vi "Auton_S2_Left_Switch.vi"   [LabVIEW 2017]
uses:
  <vilib>/Rock Robotics/WPI/Utilities/WPI_GetSetVariantRefNum.vi
  Robot Global Data.vi
  <vilib>/Rock Robotics/WPI/RobotDrive/WPI_RobotDriveArcadeDrive_Standard(NoSaturation).vi
types:
  T1 = typedef "WPI_RobotDriveDevRef.ctl" = cluster{"DevStatus":errorcluster, "Motors[]":T2[], "Square Inputs":bool, "Max Output":dbl}
  T2 = typedef "WPI_MotorControlDeviceRef.ctl" = cluster{"DeviceStatus":errorcluster, "Type":T3, "PWM":cluster{"PWM Channel":T4, "DeadBand":T5}, "CAN":cluster{"Device Number":u8, "SetOutput VI Ref":variant, "GetOutput VI Ref":variant, "Enable VI Ref":variant, "Disable VI Ref":variant, "Data":variant}, "Invert":bool, "DIO PWM":cluster{"PWM \"Enable\" Channel":T4, "DIOChannel":T6, "PWM Rate":dbl}}
  T3 = typedef "WPI_MotorControlType.ctl" = enum16{"PWM", "CAN", "DIO PWM"}
  T4 = typedef "FPGA_DIOPWMChannel.ctl" = enum8{"PWM 0", "PWM 1", "PWM 2", "PWM 3", "PWM 4", "PWM 5", "PWM 6", "PWM 7", "PWM 8", "PWM 9", "PWM MXP 0", "PWM MXP 1", "PWM MXP 2", "PWM MXP 3", "PWM MXP 4", "PWM MXP 5", "PWM MXP 6", "PWM MXP 7", "PWM MXP 8", "PWM MXP 9", "Invalid"}
  T5 = typedef "WPI_PWMDeadband.ctl" = cluster{"Name":string, "maxPositivePwm":i32, "minPositivePwm":i32, "centerPwm":i32, "maxNegativePwm":i32, "minNegativePwm":i32, "angularRange":u16}
  T6 = typedef "FPGA_DIOChannel.ctl" = enum8{"DIO 0", "DIO 1", "DIO 2", "DIO 3", "DIO 4", "DIO 5", "DIO 6", "DIO 7", "DIO 8", "DIO 9", "DIO MXP 0", "DIO MXP 1", "DIO MXP 2", "DIO MXP 3", "DIO MXP 4", "DIO MXP 5", "DIO MXP 6", "DIO MXP 7", "DIO MXP 8", "DIO MXP 9", "DIO MXP 10", "DIO MXP 11", "DIO MXP 12", "DIO MXP 13", "DIO MXP 14", "DIO MXP 15", "SPI Port CS1", "SPI Port CS2", "SPI Port CS3", "SPI Port MISO", "SPI Port MOSI", "Invalid"}
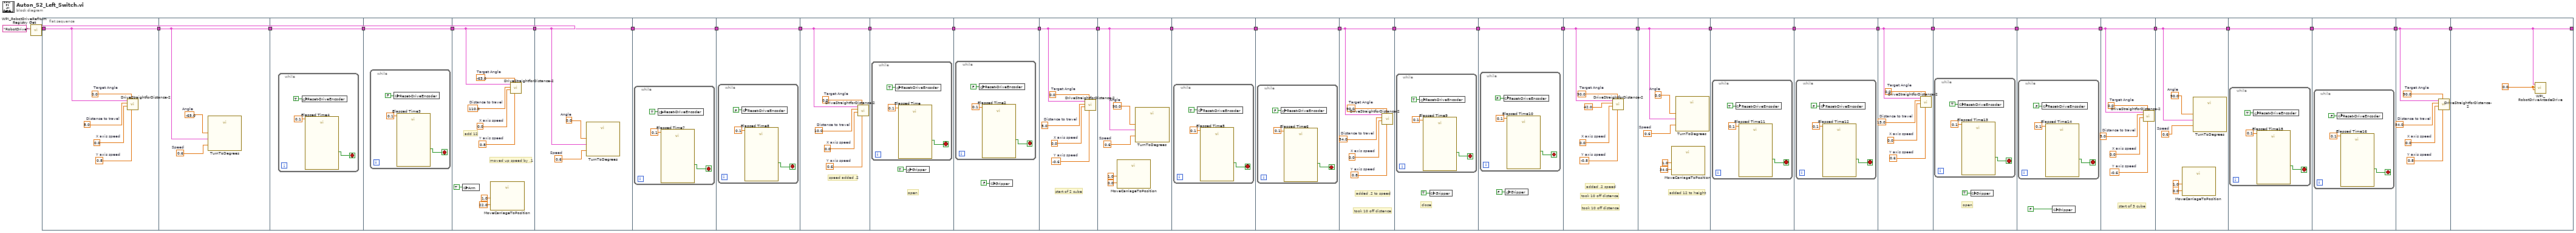
[diagram p0: block diagram]
diagram:
  n1 = call <vilib>:"WPI_RobotDriveRefNum Registry Get.vi"("refnum name"="RobotDrive") -> ("RobotDriveDevRef"=w31:T1)  [unwired: 9 in, 1 out]
  n2 = flat-sequence {
    tunnel: [w37] -> w28
    tunnel: w31 -> [w37]
    tunnel: w28 -> [w39]
    tunnel: [w39] -> w27
    tunnel: w27 -> [w41]
    tunnel: [w41] -> w29
    tunnel: w29 -> [w45]
    tunnel: [w45] -> w30
    tunnel: [w56] -> w26
    tunnel: w30 -> [w56]
    tunnel: w26 -> [w57]
    tunnel: [w57] -> w25
    tunnel: w25 -> [w60]
    tunnel: [w60] -> w24
    tunnel: w24 -> [w64]
    tunnel: [w64] -> w23
    tunnel: w23 -> [w68]
    tunnel: [w68] -> w22
    tunnel: w22 -> [w74]
    tunnel: [w74] -> w21
    tunnel: w21 -> [w79]
    tunnel: [w79] -> w20
    tunnel: w20 -> [w83]
    tunnel: [w83] -> w19
    tunnel: w19 -> [w90]
    tunnel: [w90] -> w18
    tunnel: w18 -> [w93]
    tunnel: [w93] -> w17
    tunnel: w17 -> [w97]
    tunnel: [w97] -> w16
    tunnel: w16 -> [w101]
    tunnel: [w101] -> w14
    tunnel: w14 -> [w107]
    tunnel: [w107] -> w13
    tunnel: w13 -> [w112]
    tunnel: [w112] -> w12
    tunnel: w12 -> [w116]
    tunnel: [w116] -> w15
    tunnel: w15 -> [w123]
    tunnel: [w123] -> w11
    tunnel: w11 -> [w126]
    tunnel: [w126] -> w10
    tunnel: w10 -> [w130]
    tunnel: [w130] -> w9
    tunnel: w9 -> [w134]
    tunnel: [w134] -> w8
    tunnel: w8 -> [w140]
    tunnel: [w140] -> w7
    tunnel: w7 -> [w145]
    tunnel: [w145] -> w6
    tunnel: w6 -> [w149]
    tunnel: [w149] -> w5
    tunnel: w5 -> [w154]
    tunnel: [w154] -> w4
    tunnel: w4 -> [w159]
    tunnel: [w159] -> w3
    tunnel: w3 -> [w163]
    tunnel: [w163] -> w2
    tunnel: w2 -> [w167]
    tunnel: [w167] -> w1
    tunnel: [w172] -> _
    tunnel: w1 -> [w172]
    frame #0 {
      w33 = 0.0  # Target Angle
      w34 = 0.8  # Y axis speed
      w35 = 0.0  # X axis speed
      w36 = 5.0  # Distance to travel
      n3 = call "DriveStraightforDistance-2.vi"("Y axis speed"=w34, "Target Angle"=w33, "X axis speed"=w35, "Distance to travel"=w36, "RobotDriveDevRef"=w37) -> ()  [unwired: 7 in]
    }
    frame #1 {
      w38 = -65.0  # Angle
      w40 = 0.6  # Speed
      n4 = call "TurnToDegrees.vi"("Speed"=w40, "RobotDriveDevRef"=w39, "Angle"=w38) -> ()  [unwired: 9 in]
    }
    frame #2 {
      n5 = while {
        stop <- w44 stop-if-true
        n6 = global write "Robot Global Data.vi" "Reset-DriveEncoder"(TRUE ("Reset-DriveEncoder")) -> ()
        n7 = call "Elapsed Time4"("Time Target (s)"=0.1) -> ("Time has Elapsed"=w44:bool)  [unwired: 11 in, 7 out]
      }
    }
    frame #3 {
      n8 = while {
        stop <- w48 stop-if-true
        n9 = global write "Robot Global Data.vi" "Reset-DriveEncoder"(FALSE ("Reset-DriveEncoder")) -> ()
        n10 = call "Elapsed Time3"("Time Target (s)"=0.1) -> ("Time has Elapsed"=w48:bool)  [unwired: 11 in, 7 out]
      }
    }
    frame #4 {
      w52 = -63.0  # Target Angle
      w53 = 0.8  # Y axis speed
      w54 = 0.0  # X axis speed
      w55 = 110.0  # Distance to travel
      # "add 12"
      # "moved up speed by .1"
      n11 = global write "Robot Global Data.vi" "Arm"(TRUE ("Arm")) -> ()
      n12 = call "MoveCarriageToPosition.vi"("Lift Speed"=1.0, "Target Height"=22.0) -> ()  [unwired: 10 in]
      n13 = call "DriveStraightforDistance-2.vi"("Y axis speed"=w53, "Target Angle"=w52, "X axis speed"=w54, "Distance to travel"=w55, "RobotDriveDevRef"=w56) -> ()  [unwired: 7 in]
    }
    frame #5 {
      w58 = 0.0  # Angle
      w59 = 0.6  # Speed
      n14 = call "TurnToDegrees.vi"("Speed"=w59, "RobotDriveDevRef"=w57, "Angle"=w58) -> ()  [unwired: 9 in]
    }
    frame #6 {
      n15 = while {
        stop <- w63 stop-if-true
        n16 = global write "Robot Global Data.vi" "Reset-DriveEncoder"(TRUE ("Reset-DriveEncoder")) -> ()
        n17 = call "Elapsed Time7"("Time Target (s)"=0.1) -> ("Time has Elapsed"=w63:bool)  [unwired: 11 in, 7 out]
      }
    }
    frame #7 {
      n18 = while {
        stop <- w67 stop-if-true
        n19 = global write "Robot Global Data.vi" "Reset-DriveEncoder"(FALSE ("Reset-DriveEncoder")) -> ()
        n20 = call "Elapsed Time8"("Time Target (s)"=0.1) -> ("Time has Elapsed"=w67:bool)  [unwired: 11 in, 7 out]
      }
    }
    frame #8 {
      w69 = 0.0  # Target Angle
      w70 = 0.6  # Y axis speed
      w71 = 0.0  # X axis speed
      w72 = 10.0  # Distance to travel
      # "speed added .2"
      n21 = call "DriveStraightforDistance-2.vi"("Y axis speed"=w70, "Target Angle"=w69, "X axis speed"=w71, "Distance to travel"=w72, "RobotDriveDevRef"=w68) -> ()  [unwired: 7 in]
    }
    frame #9 {
      # "open"
      n22 = while {
        stop <- w77 stop-if-true
        n23 = global write "Robot Global Data.vi" "Reset-DriveEncoder"(TRUE ("Reset-DriveEncoder")) -> ()
        n24 = call "Elapsed Time"("Time Target (s)"=0.1) -> ("Time has Elapsed"=w77:bool)  [unwired: 11 in, 7 out]
      }
      n25 = global write "Robot Global Data.vi" "Gripper"(TRUE ("Gripper")) -> ()
    }
    frame #10 {
      n26 = while {
        stop <- w82 stop-if-true
        n27 = global write "Robot Global Data.vi" "Reset-DriveEncoder"(FALSE ("Reset-DriveEncoder")) -> ()
        n28 = call "Elapsed Time2"("Time Target (s)"=0.1) -> ("Time has Elapsed"=w82:bool)  [unwired: 11 in, 7 out]
      }
      n29 = global write "Robot Global Data.vi" "Gripper"(FALSE ("Gripper")) -> ()
    }
    frame #11 {
      w84 = 0.0  # Target Angle
      w85 = -0.6  # Y axis speed
      w86 = 0.0  # X axis speed
      w87 = 5.0  # Distance to travel
      # "start of 2 cube"
      n30 = call "DriveStraightforDistance-2.vi"("Y axis speed"=w85, "Target Angle"=w84, "X axis speed"=w86, "Distance to travel"=w87, "RobotDriveDevRef"=w83) -> ()  [unwired: 7 in]
    }
    frame #12 {
      w91 = 90.0  # Angle
      w92 = 0.6  # Speed
      n31 = call "MoveCarriageToPosition.vi"("Lift Speed"=1.0, "Target Height"=0.0) -> ()  [unwired: 10 in]
      n32 = call "TurnToDegrees.vi"("Speed"=w92, "RobotDriveDevRef"=w90, "Angle"=w91) -> ()  [unwired: 9 in]
    }
    frame #13 {
      n33 = while {
        stop <- w96 stop-if-true
        n34 = global write "Robot Global Data.vi" "Reset-DriveEncoder"(TRUE ("Reset-DriveEncoder")) -> ()
        n35 = call "Elapsed Time5"("Time Target (s)"=0.1) -> ("Time has Elapsed"=w96:bool)  [unwired: 11 in, 7 out]
      }
    }
    frame #14 {
      n36 = while {
        stop <- w100 stop-if-true
        n37 = global write "Robot Global Data.vi" "Reset-DriveEncoder"(FALSE ("Reset-DriveEncoder")) -> ()
        n38 = call "Elapsed Time6"("Time Target (s)"=0.1) -> ("Time has Elapsed"=w100:bool)  [unwired: 11 in, 7 out]
      }
    }
    frame #15 {
      w102 = 90.0  # Target Angle
      w103 = 0.8  # Y axis speed
      w104 = 0.0  # X axis speed
      w105 = 54.0  # Distance to travel
      # "took 10 off distence"
      # "added .2 to speed"
      n39 = call "DriveStraightforDistance-2.vi"("Y axis speed"=w103, "Target Angle"=w102, "X axis speed"=w104, "Distance to travel"=w105, "RobotDriveDevRef"=w101) -> ()  [unwired: 7 in]
    }
    frame #16 {
      # "close"
      n40 = while {
        stop <- w110 stop-if-true
        n41 = global write "Robot Global Data.vi" "Reset-DriveEncoder"(TRUE ("Reset-DriveEncoder")) -> ()
        n42 = call "Elapsed Time9"("Time Target (s)"=0.1) -> ("Time has Elapsed"=w110:bool)  [unwired: 11 in, 7 out]
      }
      n43 = global write "Robot Global Data.vi" "Gripper"(TRUE ("Gripper")) -> ()
    }
    frame #17 {
      n44 = while {
        stop <- w115 stop-if-true
        n45 = global write "Robot Global Data.vi" "Reset-DriveEncoder"(FALSE ("Reset-DriveEncoder")) -> ()
        n46 = call "Elapsed Time10"("Time Target (s)"=0.1) -> ("Time has Elapsed"=w115:bool)  [unwired: 11 in, 7 out]
      }
      n47 = global write "Robot Global Data.vi" "Gripper"(FALSE ("Gripper")) -> ()
    }
    frame #18 {
      w118 = 90.0  # Target Angle
      w119 = -0.8  # Y axis speed
      w120 = 0.0  # X axis speed
      # "took 10 off distence"
      # "took 10 off distence"
      # "added .2 speed"
      n48 = call "DriveStraightforDistance-2.vi"("Y axis speed"=w119, "Target Angle"=w118, "X axis speed"=w120, "Distance to travel"=42.0, "RobotDriveDevRef"=w116) -> ()  [unwired: 7 in]
    }
    frame #19 {
      w124 = 0.0  # Angle
      w125 = 0.6  # Speed
      # "added 12 to height"
      n49 = call "MoveCarriageToPosition.vi"("Lift Speed"=1.0, "Target Height"=34.0) -> ()  [unwired: 10 in]
      n50 = call "TurnToDegrees.vi"("Speed"=w125, "RobotDriveDevRef"=w123, "Angle"=w124) -> ()  [unwired: 9 in]
    }
    frame #20 {
      n51 = while {
        stop <- w129 stop-if-true
        n52 = global write "Robot Global Data.vi" "Reset-DriveEncoder"(TRUE ("Reset-DriveEncoder")) -> ()
        n53 = call "Elapsed Time11"("Time Target (s)"=0.1) -> ("Time has Elapsed"=w129:bool)  [unwired: 11 in, 7 out]
      }
    }
    frame #21 {
      n54 = while {
        stop <- w133 stop-if-true
        n55 = global write "Robot Global Data.vi" "Reset-DriveEncoder"(FALSE ("Reset-DriveEncoder")) -> ()
        n56 = call "Elapsed Time12"("Time Target (s)"=0.1) -> ("Time has Elapsed"=w133:bool)  [unwired: 11 in, 7 out]
      }
    }
    frame #22 {
      w135 = 0.0  # Target Angle
      w136 = 0.6  # Y axis speed
      w137 = 0.0  # X axis speed
      w138 = 15.0  # Distance to travel
      n57 = call "DriveStraightforDistance-2.vi"("Y axis speed"=w136, "Target Angle"=w135, "X axis speed"=w137, "Distance to travel"=w138, "RobotDriveDevRef"=w134) -> ()  [unwired: 7 in]
    }
    frame #23 {
      # "open"
      n58 = while {
        stop <- w143 stop-if-true
        n59 = global write "Robot Global Data.vi" "Reset-DriveEncoder"(TRUE ("Reset-DriveEncoder")) -> ()
        n60 = call "Elapsed Time13"("Time Target (s)"=0.1) -> ("Time has Elapsed"=w143:bool)  [unwired: 11 in, 7 out]
      }
      n61 = global write "Robot Global Data.vi" "Gripper"(TRUE ("Gripper")) -> ()
    }
    frame #24 {
      n62 = while {
        stop <- w148 stop-if-true
        n63 = global write "Robot Global Data.vi" "Reset-DriveEncoder"(FALSE ("Reset-DriveEncoder")) -> ()
        n64 = call "Elapsed Time14"("Time Target (s)"=0.1) -> ("Time has Elapsed"=w148:bool)  [unwired: 11 in, 7 out]
      }
      n65 = global write "Robot Global Data.vi" "Gripper"(FALSE ("Gripper")) -> ()
    }
    frame #25 {
      w150 = 0.0  # Target Angle
      w151 = -0.6  # Y axis speed
      w152 = 0.0  # X axis speed
      w153 = 5.0  # Distance to travel
      # "start of 3 cube"
      n66 = call "DriveStraightforDistance-2.vi"("Y axis speed"=w151, "Target Angle"=w150, "X axis speed"=w152, "Distance to travel"=w153, "RobotDriveDevRef"=w149) -> ()  [unwired: 7 in]
    }
    frame #26 {
      w157 = 90.0  # Angle
      w158 = 0.6  # Speed
      n67 = call "MoveCarriageToPosition.vi"("Lift Speed"=1.0, "Target Height"=0.0) -> ()  [unwired: 10 in]
      n68 = call "TurnToDegrees.vi"("Speed"=w158, "RobotDriveDevRef"=w154, "Angle"=w157) -> ()  [unwired: 9 in]
    }
    frame #27 {
      n69 = while {
        stop <- w162 stop-if-true
        n70 = global write "Robot Global Data.vi" "Reset-DriveEncoder"(TRUE ("Reset-DriveEncoder")) -> ()
        n71 = call "Elapsed Time15"("Time Target (s)"=0.1) -> ("Time has Elapsed"=w162:bool)  [unwired: 11 in, 7 out]
      }
    }
    frame #28 {
      n72 = while {
        stop <- w166 stop-if-true
        n73 = global write "Robot Global Data.vi" "Reset-DriveEncoder"(FALSE ("Reset-DriveEncoder")) -> ()
        n74 = call "Elapsed Time16"("Time Target (s)"=0.1) -> ("Time has Elapsed"=w166:bool)  [unwired: 11 in, 7 out]
      }
    }
    frame #29 {
      w168 = 90.0  # Target Angle
      w169 = 0.8  # Y axis speed
      w170 = 0.0  # X axis speed
      w171 = 54.0  # Distance to travel
      n75 = call "DriveStraightforDistance-2.vi"("Y axis speed"=w169, "Target Angle"=w168, "X axis speed"=w170, "Distance to travel"=w171, "RobotDriveDevRef"=w167) -> ()  [unwired: 7 in]
    }
    frame #30 {
      w173 = 0.0 ("X axis value")
      n76 = call-poly <vilib>:"WPI_RobotDriveArcadeDrive.vi"("Y axis value"=w173, "X axis value"=w173, "RobotDriveDevRef"=w172) -> ()  [unwired: 6 in, 3 out]
    }
  }
